vi "SPI Engine. SPICore.vi"(6 "Ready for Output":bool, 9 "Input Valid":bool, 10 "SPI Information In":T1, 11 "SPI DIO Input":T4) -> (1 "Output Valid":bool, 2 "SPI Output Data":T2, 3 "SPI DIO Output":T3, 4 "Ready For Input":bool, 5 "Chip Select ID":u8)   [LabVIEW 2014]
doc: "This VI performs the actual SPI Transactions. It wraps the SPI Core with added functionality of 4-Wire Handshake"
uses:
  user.lib/_NI SPI IP/FPGA/Controllers/Public/Spi Master Inputs.ctl
  user.lib/_NI SPI IP/FPGA/Controllers/Public/Spi Master Outputs.ctl
  Controls/SPI Response Information.ctl
  Controls/SPI Transaction Packet.ctl
  user.lib/_NI SPI IP/FPGA/Controllers/NI SPI IP (FPGA).lvlib
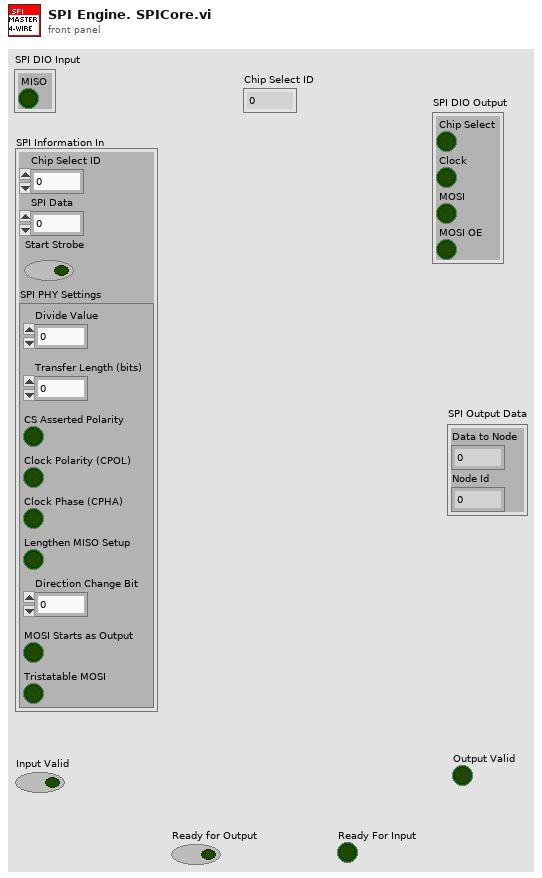
[diagram p1: front panel]
types:
  T1 = typedef "SPI Transaction Packet.ctl" = cluster{"Chip Select ID":u8, "SPI Data":u64, "Start Strobe":bool, "SPI PHY Settings":cluster{"Divide Value":u8, "Transfer Length (bits)":u8, "CS Asserted Polarity":bool, "Clock Polarity (CPOL)":bool, "Clock Phase (CPHA)":bool, "Lengthen MISO Setup":bool, "Direction Change Bit":u8, "MOSI Starts as Output":bool, "Tristatable MOSI":bool}}
  T2 = typedef "SPI Response Information.ctl" = cluster{"Data to Node":u64, "Node Id":u16}
  T3 = typedef "NI SPI IP (FPGA).lvlib/Spi Master Outputs.ctl" = cluster{"Chip Select":bool, "Clock":bool, "MOSI":bool, "MOSI OE":bool}
  T4 = typedef "NI SPI IP (FPGA).lvlib/Spi Master Inputs.ctl" = cluster{"MISO":bool}
  T5 = cluster{"Divide Value":u8, "Transfer Length (bits)":u8, "CS Asserted Polarity":bool, "Clock Polarity (CPOL)":bool, "Clock Phase (CPHA)":bool, "Lengthen MISO Setup":bool, "Direction Change Bit":u8, "MOSI Starts as Output":bool, "Tristatable MOSI":bool}
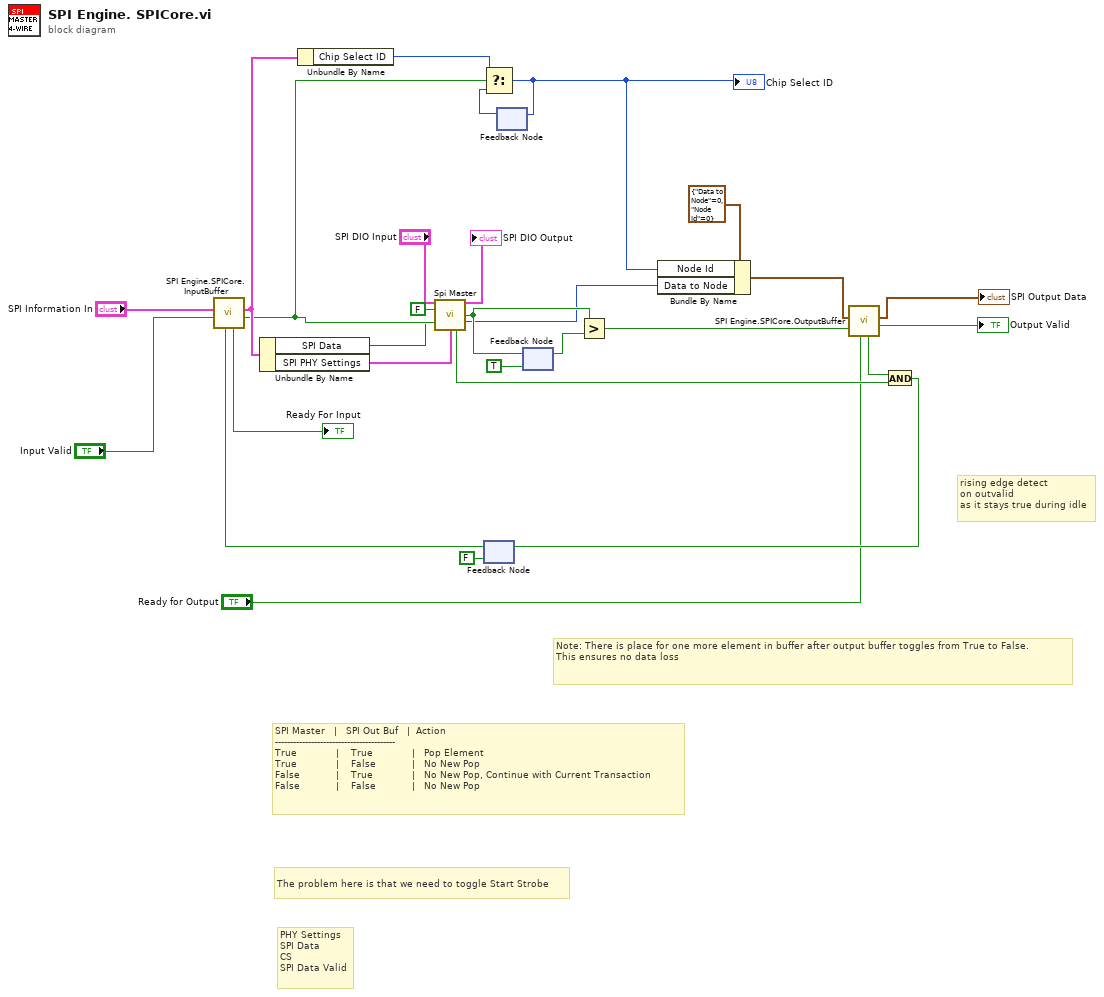
[diagram p0: block diagram]
diagram:
  # "rising edge detect\non outvalid\nas it stays true during idle"
  # "PHY Settings\nSPI Data\nCS\nSPI Data Valid"
  # "The problem here is that we need to toggle Start Strobe"
  # "Note: There is place for one more element in buffer after output buffer toggles from True to False.\nThis ensures no data loss"
  # "SPI Master   |   SPI Out Buf   |  Action\n----------------------------------------\nTrue             |    True             |   Pop Element\nTrue             |    False            |   No New Pop \nFalse            |    True             |   No New Pop, Continue with Current Transaction\nFalse            |    False            |   No New Pop"
  n1 = feedback #1(FALSE) -> (w25:bool)
  n2 = call "SPI Engine.SPICore.InputBuffer.vi"("Ready for Output"=w25, "Input Valid"="Input Valid", "SPI Information In"="SPI Information In") -> ("Output Data"=w2:bool, "SPI Information Out"=w18:T1, "Ready For Input"=→"Ready For Input":bool)  [unwired: 6 in]
  n3 = Unbundle By Name(w18) -> ("SPI Data"=w1:u64, "SPI PHY Settings"=w17:T5)
  n4 = Unbundle By Name(w18) -> ("Chip Select ID"=w10:u8)
  n5 = call "Spi Master.vi"("spi input"="SPI DIO Input", "manual assert chip select"=FALSE, "start strobe"=w2, "data to write"=w1, "spi transfer settings"=w17) -> ("spi output"=→"SPI DIO Output":T3, "read data valid"=w11:bool, "read data"=w7:u64, "ready for input"=w27:bool)  [unwired: 7 in]
  n6 = feedback #2() -> (w9:u8)  [unwired: 1 in]
  n7 = Select(t=w10, s=w2, f=w9) -> (s? t:f=w6:u8)
  "Chip Select ID" <- w6
  n8 = feedback-in #2(w6) -> ()
  n9 = feedback-in #3(w11) -> ()
  n10 = feedback #3(TRUE ("read data valid")) -> (w14:bool)
  n11 = Greater?(x=w11, y=w14) -> (0:w3:bool)
  n12 = Bundle By Name(cluster=T2 {"Data to Node"=0, "Node Id"=0} ("SPI Response"), "Node Id"=w6, "Data to Node"=w7) -> (w4:T2)
  n13 = call "SPI Engine.SPICore.OutputBuffer.vi"("Ready for Output"="Ready for Output", "Input Valid"=w3, "Input Data"=w4) -> ("Output Valid"=→"Output Valid":bool, "Output Data"=→"SPI Output Data":T2, "Ready For Input"=w28:bool)  [unwired: 6 in]
  n14 = And(x=w28, y=w27) -> (x .and. y?=w26:bool)
  n15 = feedback-in #1(w26) -> ()
